vi "Compute DistanceToTarget2.vi"(8 "Calibrated":bool, 9 "Camera Type":T6, 10 "Line":T4, 11 "Image Src":T5) -> (1 "Edges":cluster{"X":sgl, "Y":sgl}[](array[cluster]), 2 "Distance (ft)":dbl, 3 "Image Dst Out":T5)   [LabVIEW 2016]
doc: "Using the camera lens information and the real world size of the target, use trig and ratios to determine the distance to the target. Also returns the location relative to the image center in a (-1 , 1) coordinate system that may be useful for steering the robot."
uses:
  Camera Types.ctl
  <vilib>/vision/Image Controls.llb/IMAQ Image.ctl
  <vilib>/vision/Measure.llb/Edge New.ctl
  <vilib>/vision/Measure.llb/Edge Options.ctl
  <vilib>/vision/Measure.llb/Edge Polarity.ctl
  <vilib>/vision/NI_Vision_Development_Module.lvlib
panel:
  in  "Edge Options":T1={"Edge Polarity"=0, "Kernel Size"=3, "Width"=3, "Minimum Edge Strength"=30.0, "Interpolation Type"=enum."Bilinear Fixed", "Data Processing Method"=enum."Average"} {"Edge Polarity" items=["All Edges", "Rising Edges", "Falling Edges"]; "Minimum Edge Strength" format="%.2f"; "Width" step=2; "Kernel Size" step=2}
  out "lengths":dbl[](array[numeric])
  out "Edge Information":T3[](array[typedef]) {"Distance (Real-World)" format="%.2f"; "Location (Real-World)"."Y" format="%.2g"; "Location (Real-World)"."X" format="%.2f"; "Noise" format="%.2f"; "Location (Pixel)"."Y" format="%.2g"; "Location (Pixel)"."X" format="%.2f"; "Strength" format="%.2f"; "Distance (Pixel)" format="%.2f"}
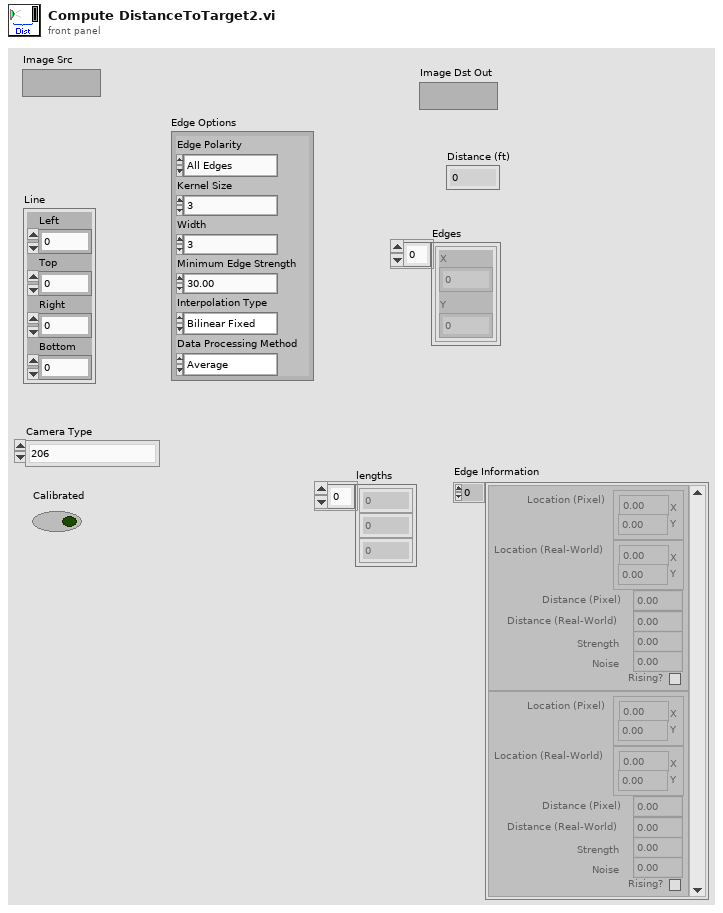
[diagram p1: front panel]
types:
  T1 = typedef "Edge Options.ctl" = cluster{"Edge Polarity":T2, "Kernel Size":u32, "Width":u32, "Minimum Edge Strength":sgl, "Interpolation Type":enum32{"Zero Order", "Bilinear", "Quadratic", "Cubic", "Bilinear Fixed"}, "Data Processing Method":enum32{"Average", "Median"}}
  T2 = typedef "Edge Polarity.ctl" = u32
  T3 = typedef "Edge New.ctl" = cluster{"Location (Pixel)":cluster{"X":sgl, "Y":sgl}, "Location (Real-World)":cluster{"X":sgl, "Y":sgl}, "Distance (Pixel)":dbl, "Distance (Real-World)":dbl, "Strength":dbl, "Noise":dbl, "Rising?":bool}
  T4 = cluster{"Left":dbl, "Top":dbl, "Right":dbl, "Bottom":dbl}
  T5 = typedef "IMAQ Image.ctl" = refnum<image>
  T6 = typedef "Camera Types.ctl" = enum16{"206", "1011", "1013", "MS HD3000 square", "MS HD3000 640x480"}
  T7 = enum16{"Get First Edge", "Get First + Last Edge", "Get All Edges", "Get Best Edge"}
  T8 = typedef "ROI Descriptor" = cluster{"Global Rectangle":i32[], "Contours":cluster{"ID":enum32{"External", "Internal"}, "Type":u32, "Coordinates":i32[]}[]}
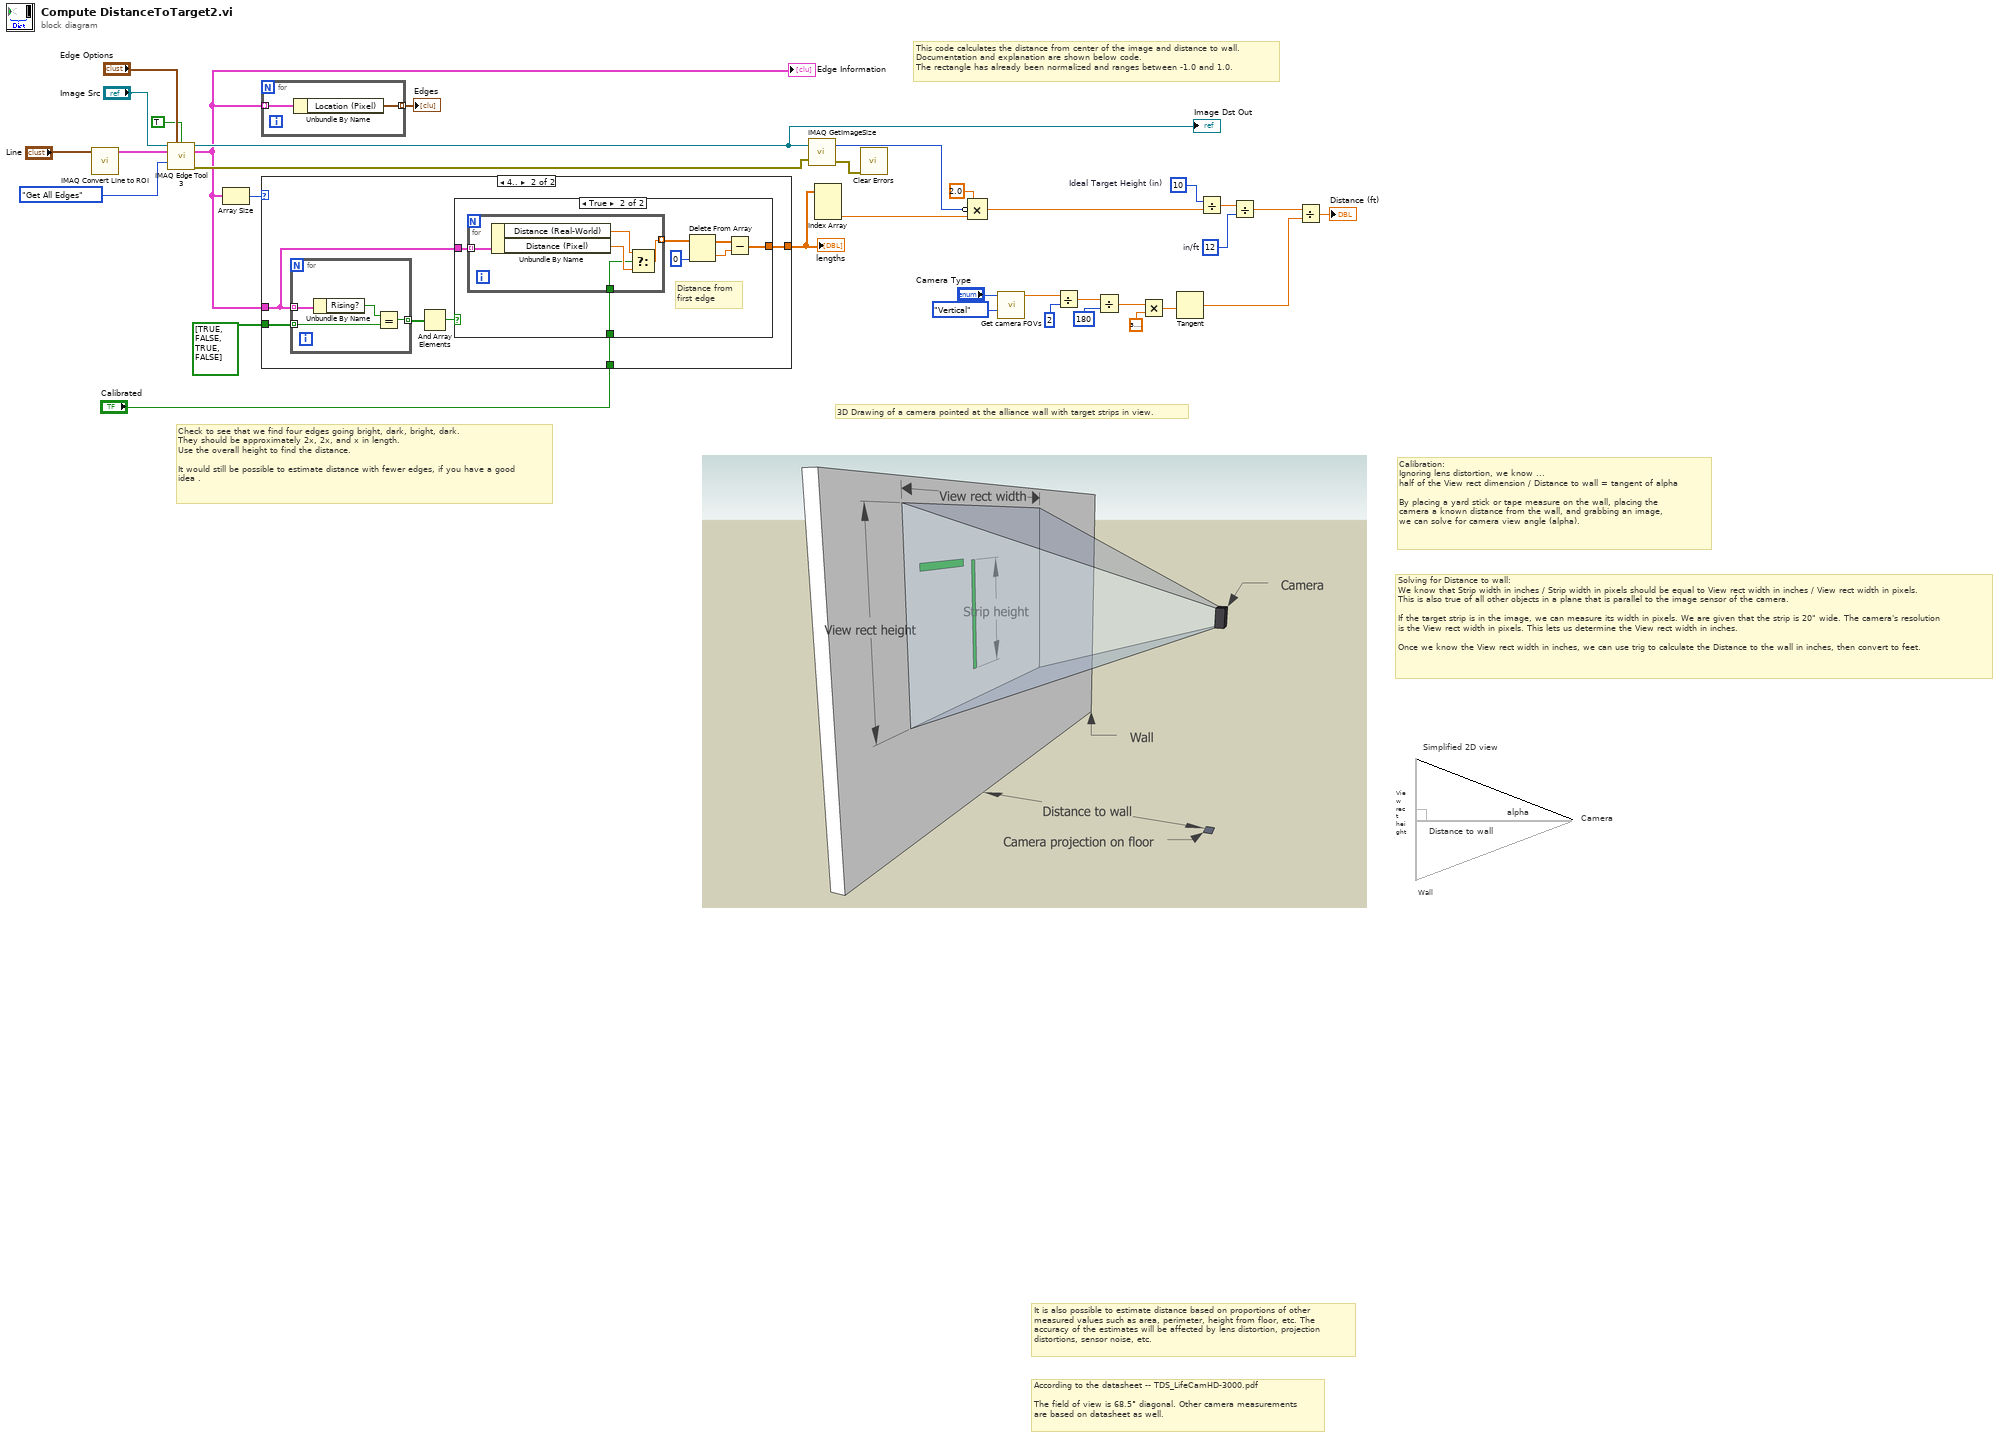
[diagram p0: block diagram]
diagram:
  w21 = 10  # Ideal Target Height (in)
  w28 = 12  # in/ft
  # "Check to see that we find four edges going bright, dark, bright, dark.\nThey should be approximately 2x, 2x, and x in length.\nUse the overall height to find the distance.\n\nIt would still be possible to estimate distance with fewer edges, if you have a good\nidea ."
  # "It is also possible to estimate distance based on proportions of other\nmeasured values such as area, perimeter, height from floor, etc. The\naccuracy of the estimates will be affected by lens distortion, projection\ndistortions, sensor noise, etc."
  # "According to the datasheet -- TDS_LifeCamHD-3000.pdf\n\nThe field of view is 68.5° diagonal. Other camera measurements\nare based on datasheet as well."
  # "Wall"
  # "Camera"
  # "Simplified 2D view"
  # "Solving for Distance to wall:\nWe know that Strip width in inches / Strip width in pixels should be equal to View rect width in inches / View rect width in pixels.\nThis is also true of all other objects in a plane that is parallel to the image sensor of the camera.\n\nIf the target strip is in the image, we can measure its width in pixels. We are given that the strip is 20\" wide. The camera's resolution\nis the View rect width in pixels. This lets us determine the View rect width in inches.\n\nOnce we know the View rect width in inches, we can use trig to calculate the Distance to the wall in inches, then convert to feet."
  # "3D Drawing of a camera pointed at the alliance wall with target strips in view."
  # "Distance to wall"
  # "View rect height"
  # "alpha"
  # "Calibration:\nIgnoring lens distortion, we know ...\nhalf of the View rect dimension / Distance to wall = tangent of alpha\n\nBy placing a yard stick or tape measure on the wall, placing the\ncamera a known distance from the wall, and grabbing an image,\nwe can solve for camera view angle (alpha)."
  # "This code calculates the distance from center of the image and distance to wall.\nDocumentation and explanation are shown below code.\nThe rectangle has already been normalized and ranges between -1.0 and 1.0."
  n1 = call "IMAQ Convert Line to ROI"("Line"="Line") -> ("ROI Descriptor"=w18:T8)  [unwired: 8 in, 1 out]
  n2 = call "IMAQ Edge Tool 3"("Image"="Image Src", "Edge Options"="Edge Options", "Optimized Mode"=TRUE, "ROI Descriptor"=w18, "Process"=T7."Get All Edges") -> ("Image (duplicate)"=w3:T5, "Edge Information"=w2:T3[], "error out"=w7:errorcluster)  [unwired: 6 in, 2 out]
  "Image Dst Out" <- w3
  "Edge Information" <- w2
  n3 = Array Size(array=w2) -> (size(s)=w14:i32)
  n4 = for {
    tunnel: w2 -> [w36] mode=indexing
    tunnel: [w35] -> w1 mode=indexing
    n5 = Unbundle By Name(w36) -> ("Location (Pixel)"=w35:cluster{"X":sgl, "Y":sgl})
  }
  "Edges" <- w1
  n6 = case shown="4.." w14 {
    tunnel: w2 -> [_ w39]
    tunnel: bool[] [TRUE, FALSE, TRUE, FALSE] -> [_ w42]
    tunnel: [_ w38] -> w12
    tunnel: "Calibrated" -> [_ w37]
    frame 0, Default {
    }
    frame 4.. {
      n7 = for {
        tunnel: w39 -> [w58] mode=indexing
        tunnel: w42 -> [w56] mode=indexing
        tunnel: [w55] -> w41 mode=indexing
        n8 = Unbundle By Name(w58) -> ("Rising?"=w57:bool)
        n9 = Equal?(x=w57, y=w56) -> (x = y?=w55:bool)
      }
      n10 = And Array Elements(Boolean array=w41) -> (logical AND=w40:bool)
      n11 = case shown="True" w40 {
        tunnel: w39 -> [_ w49]
        tunnel: [_ w45] -> w38
        tunnel: w37 -> [_ w43]
        frame False {
        }
        frame True {
          # "Distance from\nfirst edge"
          n12 = for {
            tunnel: w49 -> [w54] mode=indexing
            tunnel: [w52] -> w48 mode=indexing
            tunnel: w43 -> [w50]
            n13 = Unbundle By Name(w54) -> ("Distance (Real-World)"=w53:dbl, "Distance (Pixel)"=w51:dbl)
            n14 = Select(t=w53, s=w50, f=w51) -> (s? t:f=w52:dbl)
          }
          n15 = Delete From Array(array=w48, index=0) -> (deleted portion=w44:dbl, array with subset deleted=w46:dbl[])  [unwired: 1 in]
          n16 = Subtract(x=w46, y=w44) -> (x-y=w45:dbl[])
        }
      }
    }
  }
  "lengths" <- w12
  n17 = call "IMAQ GetImageSize"("Image"=w3, "error in (no error)"=w7) -> ("Y Resolution"=w8:i32, "error out"=w6:errorcluster)  [unwired: 2 in, 1 out]
  n18 = Index Array(array=w12) -> (element #3=w10:dbl)  [unwired: 3 in, 2 out]
  n19 = call <vilib>:"Clear Errors.vi"("error in (no error)"=w6) -> ()  [unwired: 5 in, 2 out]
  n20 = Compound Arithmetic op=MULTIPLY(2.0, invert w8, w10) -> (w9:dbl)
  n21 = call "Get camera FOVs.vi"("Type"=enum16{"Horizontal", "Vertical", "Diagonal"}."Vertical" ("Angle"), "Camera Type"="Camera Type") -> ("FOV"=w23:dbl)  [unwired: 8 in, 1 out]
  n22 = Divide(x=w23, y=2) -> (x/y=w31:dbl)
  n23 = Divide(x=w31, y=180) -> (x/y=w30:dbl)
  n24 = Multiply(x=w30, y=3.141592653589793) -> (x*y=w32:dbl)
  n25 = Tangent(1:w32) -> (0:w27:dbl)
  n26 = Divide(x=w21, y=w9) -> (x/y=w25:dbl)
  n27 = Divide(x=w25, y=w28) -> (x/y=w24:dbl)
  n28 = Divide(x=w24, y=w27) -> (x/y=→"Distance (ft)":dbl)
